vi "Read Potentiostat Voltage.vi"(0 "VISA Refnum in":refnum<visa-resource-name>, 2 "Flush after read":bool=TRUE, 3 "error in (no error)":errorcluster) -> (7 "VISA Refnum out":refnum<visa-resource-name>, 8 "Voltage":dbl, 10 "error out":errorcluster)   [LabVIEW 2019]
uses:
  <vilib>/Utility/error.llb/Error Cluster From Error Code.vi
  <vilib>/regexp/Match Regular Expression.xnode
  <vilib>/ErrorRing/Error Ring.xnode
panel:
  out "String":string
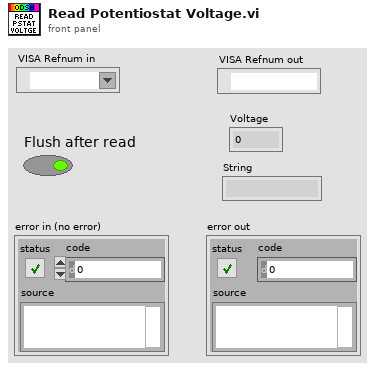
[diagram p1: front panel]
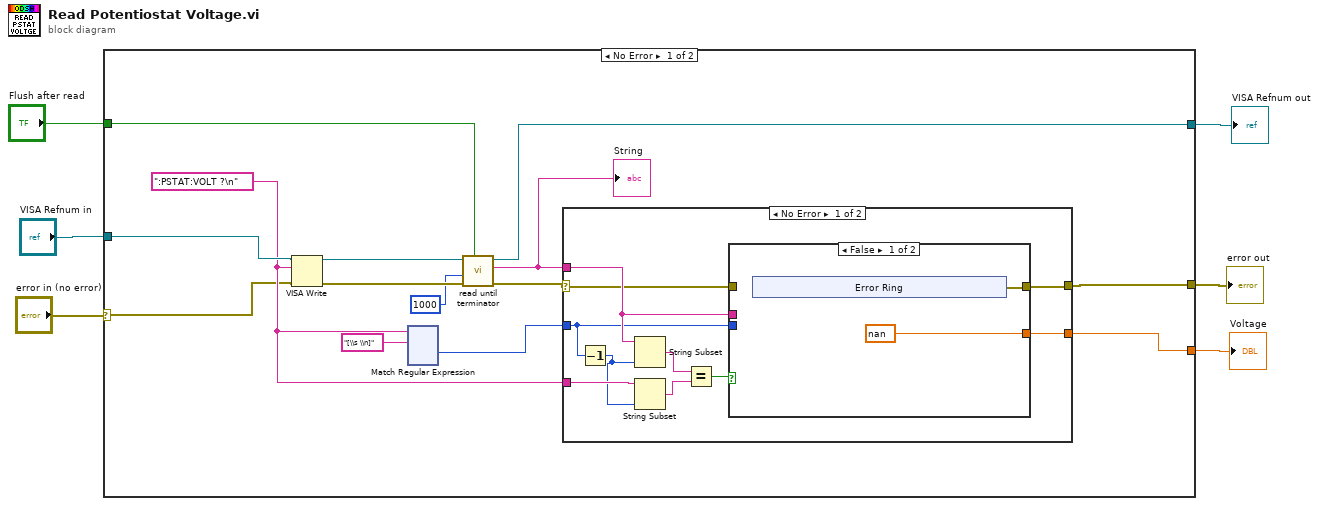
[diagram p0: block diagram]
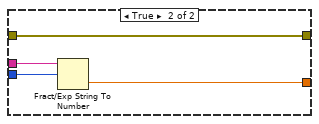
[diagram p2: hidden frame]
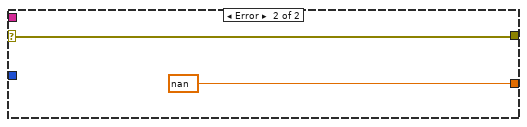
[diagram p3: hidden frame]
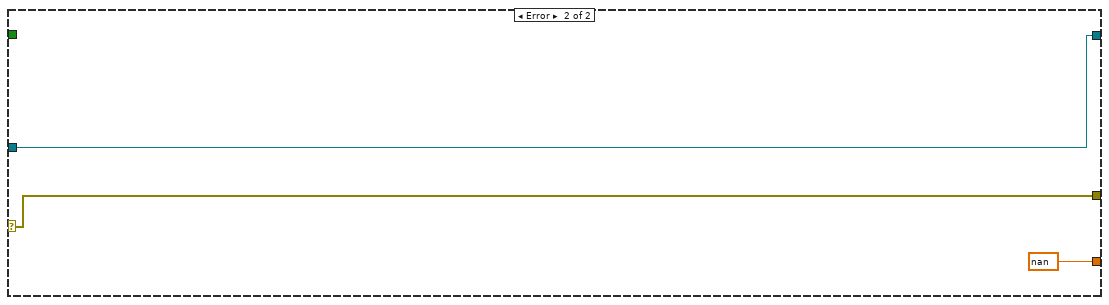
[diagram p4: hidden frame]
diagram:
  n1 = case shown="No Error" "error in (no error)" {
    selector: "error in (no error)" -> [w8 w160]
    tunnel: "VISA Refnum in" -> [w20 w159]
    tunnel: [w17 w159] -> w5
    tunnel: [w15 nan] -> w4
    tunnel: [w13 w160] -> w3
    tunnel: "Flush after read" -> [w7 _]
    frame No Error {
      w9 = ":PSTAT:VOLT ?\n" ("buffer d'écriture")
      n2 = VISA Write(VISA resource name=w20, write buffer=w9, error in (no error)=w8) -> (VISA resource name out=w19:refnum<visa-resource-name>, error out=w18:errorcluster)  [unwired: 1 out]
      n3 = xnode "Match Regular Expression"("input string"=w9, "regular expression"="[\\s \\n]") -> ("offset past match"=w10:i32)  [unwired: 4 in, 4 out]
      n4 = call "read until terminator.vi"("Flush after read"=w7, "error in (no error)"=w18, "Timeout (ms)"=1000, "VISA Refnum in"=w19) -> ("error out"=w14:errorcluster, "String"=w12:string, "VISA Refnum out"=w17:refnum<visa-resource-name>)  [unwired: 5 in]
      "String" <- w12
      n5 = case shown="No Error" w14 {
        selector: w14 -> [w138 w156]
        tunnel: w12 -> [w142 _]
        tunnel: [w144 nan] -> w15
        tunnel: [w137 w156] -> w13
        tunnel: w10 -> [w136 _]
        tunnel: w9 -> [w143 _]
        frame No Error {
          n6 = Decrement(x=w136) -> (x-1=w135:i32)
          n7 = String Subset(string=w142, length (rest)=w135) -> (substring=w141:string)  [unwired: 1 in]
          n8 = String Subset(string=w143, length (rest)=w135) -> (substring=w140:string)  [unwired: 1 in]
          n9 = Equal?(x=w141, y=w140) -> (x = y?=w139:bool)
          n10 = case shown="False" w139 {
            tunnel: [nan w155] -> w144
            tunnel: w142 -> [_ w154]
            tunnel: w136 -> [_ w153]
            tunnel: w138 -> [_ w152]
            tunnel: [w145 w152] -> w137
            frame False {
              n11 = xnode "Error Ring"() -> ("error out"=w145:errorcluster)
            }
            frame True {
              n12 = Fract/Exp String To Number(string=w154, offset=w153) -> (number=w155:dbl)  [unwired: 2 in, 1 out]
            }
          }
        }
        frame Error {
        }
      }
    }
    frame Error {
    }
  }
  "error out" <- w3
  "VISA Refnum out" <- w5
  "Voltage" <- w4
